vi "Check if Build Assets Exists.vi"(8 "error in":errorcluster, 11 "project ref":refnum<vi>) -> (0 "error out":errorcluster, 3 "build assests exists?":bool)   [LabVIEW 2021, in "MeasurementService Editor.lvlib"]
uses:
  MeasurementService Editor.lvlib
  7954e2c4-fa36-4556-a137-9531e1e52501.vi
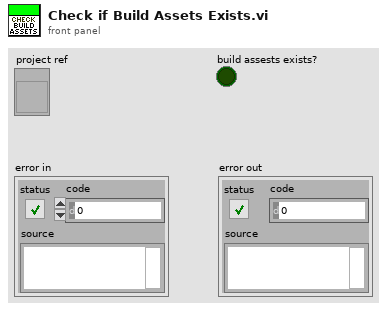
[diagram p1: front panel]
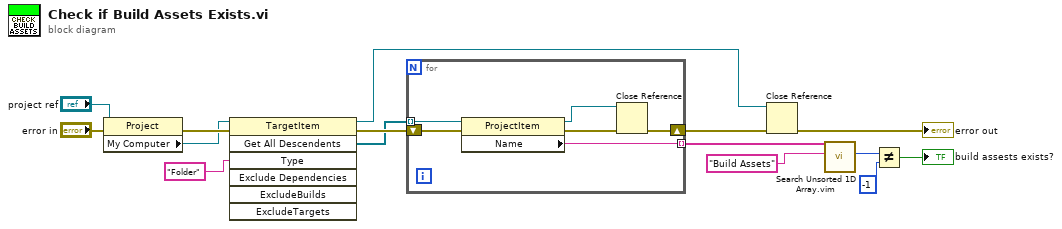
[diagram p0: block diagram]
diagram:
  n1 = property class="Project"(reference="project ref", error in="error in") -> (error out=w15:errorcluster, "My Computer"=w14:refnum<vi>)  [unwired: 1 out]
  n2 = invoke class="TargetItem" method="Get All Descendents"(reference=w14, error in=w15, "Type"="Folder") -> (reference out=w1:refnum<vi>, error out=w9:errorcluster, "All Descendents"=w8:refnum<vi>[])  [unwired: 4 in, 4 out]
  n3 = for {
    tunnel: w8 -> [w19] mode=indexing
    shift-right: [w17] -> w3
    shift-left: w9 -> [w20]
    tunnel: [w16] -> w6 mode=indexing
    n4 = property class="ProjectItem"(reference=w19, error in=w20) -> (reference out=w18:refnum<vi>, error out=w21:errorcluster, "Name"=w16:string)
    n5 = Close Reference(reference=w18, error in (no error)=w21) -> (error out=w17:errorcluster)
  }
  n6 = Close Reference(reference=w1, error in (no error)=w3) -> (error out=→"error out":errorcluster)
  n7 = call "Search Unsorted 1D Array.vim"("element"="Build Assets", "unsorted 1D array"=w6) -> ("index of element"=w12:i32)  [unwired: 9 in]
  n8 = Not Equal?(x=w12, y=-1) -> (x != y?=→"build assests exists?":bool)
